vi "Set SPI Engine SCLK Divisor.vi"(8 "error in":errorcluster, 9 "Set? (T)":bool=TRUE, 10 "SPI Engine Clock Divisor":u8=4 min=4, 11 "SPI Engine Resources":T1={"To SPI Engine Data FIFO"="DLU To SPI Engine Data", "From SPI Engine Data FIFO"="SPI Engine to DLU Data", "Data to SPI Engine (Cache) Register"="Data to SPI Engine (Cache)", "SPI Settings to SPI Engine (Cache) Register"="SPI PHY Settings to SPI Engine (Cache)"}) -> (0 "error out":errorcluster, 2 "Actual Divisor":u8, 3 "SPI Engine Resources":T1={"To SPI Engine Data FIFO"="DLU To SPI Engine Data", "From SPI Engine Data FIFO"="SPI Engine to DLU Data", "Data to SPI Engine (Cache) Register"="Data to SPI Engine (Cache)", "SPI Settings to SPI Engine (Cache) Register"="SPI PHY Settings to SPI Engine (Cache)"})   [LabVIEW 2015]
doc: "This VI configures the clock divisor used to generate SCLK. The divisor will divide the clock driving the SPI Engine to generate the resulting SCLK signal. For example, a SPI Engine running in a 120MHz SCTL with a divisor of 12 will yield a 10MHz SCLK."
uses:
  Controls/SPI Engine Resources.ctl
  <vilib>/rvi/DataTransferAndStorage/Container/Common/niFpgaContainerExecOnDevCompGetState.vi
  <vilib>/rvi/Emulation/niFpgaEmulationIsFPGAContextNoSignature.vi
  <vilib>/rvi/DataTransferAndStorage/Container/Common/niFpgaContainerGetUniqueNameForEmu.vi
  <vilib>/rvi/Memory/Memory_Emulation/niFpgaMemoryEmulationCacheClearOnFirstRun.vi
  <vilib>/rvi/Memory/Memory_Emulation/nirvimemoryEmulationManagerCache_MakeExclusive.vi
  <vilib>/rvi/Memory/Memory_Emulation/niFpgaMemoryEmulationValidateCache.vi
  <vilib>/rvi/Memory/Memory_Emulation/nirvimemoryEmulationManagerCache_InsertValue.vi
  <vilib>/Utility/error.llb/Clear Errors.vi
  <vilib>/rvi/Memory/Memory_Emulation/nirvimemoryEmulationManagerCache_ReleaseExclusive.vi
  <vilib>/rvi/Memory/Memory_Emulation/nirvimemoryEmulationManagerCache_GetValue.vi
  <vilib>/rvi/Memory/Memory_Emulation/nirvimemoryEmulationManagerCache_SetValue.vi
  <vilib>/rvi/Emulation/niFpgaProcessEmulError.vi
  <vilib>/rvi/Emulation/niFpgaSctlEmulationGetInTimedLoop.vi
  <vilib>/rvi/DataTransferAndStorage/Container/XNode/niFpgaContainer.xnode
  <vilib>/rvi/DataTransferAndStorage/Register/Emulation/niFpgaRegisterEmulationRefIn.vi
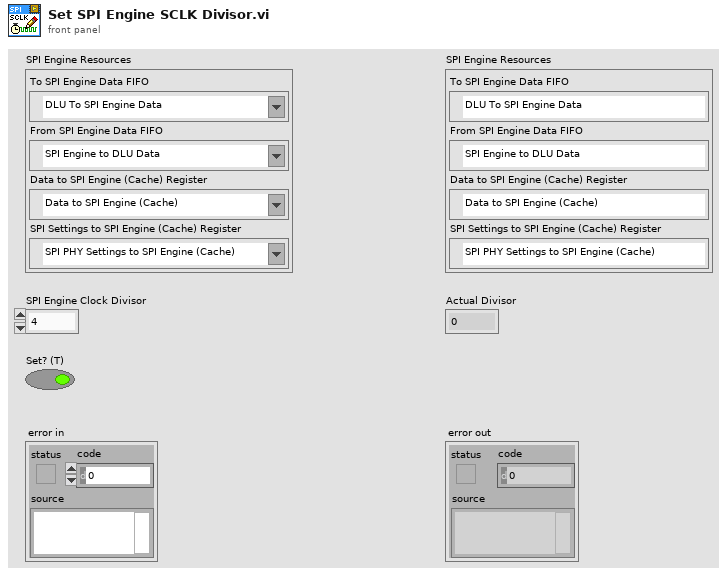
[diagram p1: front panel]
types:
  T1 = typedef "SPI Engine Resources.ctl" = cluster{"To SPI Engine Data FIFO":refnum<k21>, "From SPI Engine Data FIFO":refnum<k21>, "Data to SPI Engine (Cache) Register":refnum<k21>, "SPI Settings to SPI Engine (Cache) Register":refnum<k21>}
  T2 = cluster{"Chip Select ID":u8, "SPI PHY Settings":cluster{"Divide Value":u8, "Transfer Length (bits)":u8, "CS Asserted Polarity":bool, "Clock Polarity (CPOL)":bool, "Clock Phase (CPHA)":bool, "Lengthen MISO Setup":bool, "Direction Change Bit":u8, "MOSI Starts as Output":bool, "Tristatable MOSI":bool}}
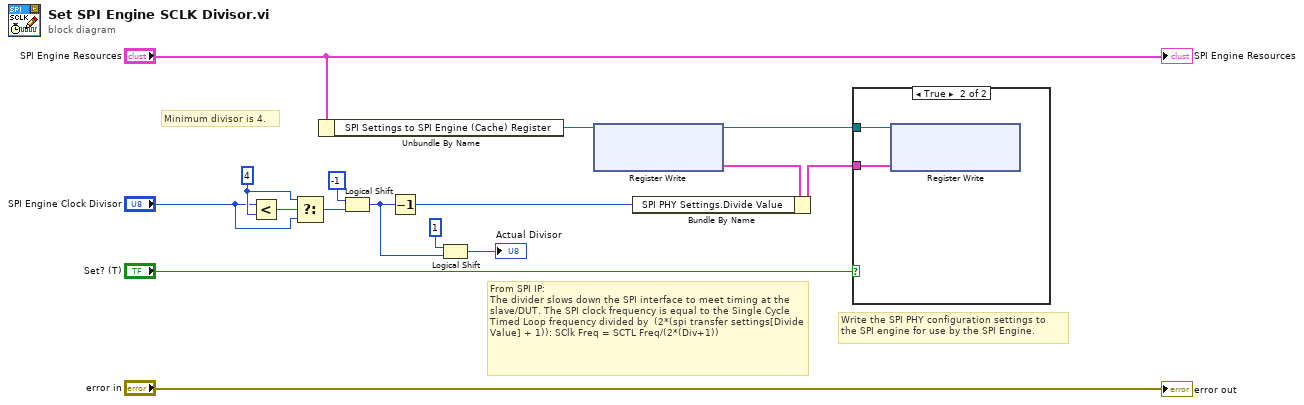
[diagram p0: block diagram]
diagram:
  w7 = u8 4 ("y")
  # "Minimum divisor is 4."
  # "From SPI IP:\nThe divider slows down the SPI interface to meet timing at the slave/DUT. The SPI clock frequency is equal to the Single Cycle Timed Loop frequency divided by  (2*(spi transfer settings[Divide Value] + 1)): SClk Freq = SCTL Freq/(2*(Div+1))"
  # "Write the SPI PHY configuration settings to\nthe SPI engine for use by the SPI Engine."
  n1 = Less?(x="SPI Engine Clock Divisor", y=w7) -> (x < y?=w8:bool)
  n2 = Select(t=w7, s=w8, f="SPI Engine Clock Divisor") -> (s? t:f=w5:u8)
  n3 = Unbundle By Name("SPI Engine Resources") -> ("SPI Settings to SPI Engine (Cache) Register"=w14:refnum<k21>)
  n4 = Logical Shift(y=i16 -1 ("n"), x=w5) -> (x << y=w2:u8)
  n5 = Decrement(x=w2) -> (x-1=w11:u8)
  n6 = Logical Shift(y=i16 1 ("n"), x=w2) -> (x << y=→"Actual Divisor":u8)
  n7 = xnode ("Register Write")("Register In"=w14) -> ("Data"=w9:T2, "Register Out"=w13:refnum<k21>)
  n8 = Bundle By Name(cluster=w9, "SPI PHY Settings.Divide Value"=w11) -> (w10:T2)
  n9 = case shown="True" "Set? (T)" {
    tunnel: w13 -> [_ w18]
    tunnel: w10 -> [_ w17]
    frame False {
    }
    frame True {
      n10 = xnode ("Register Write")("Data"=w17, "Register In"=w18) -> ()  [unwired: 1 out]
    }
  }
  "error out" <- "error in"
  "SPI Engine Resources" <- "SPI Engine Resources"
